vi "Upload File.vi"(8 "error in (no error)":errorcluster, 9 "Relative Path":string, 10 "Local File":path, 11 "Artifactory in":refnum<class "Artifactory.lvclass">) -> (0 "error out":errorcluster, 3 "Artifactory out":refnum<class "Artifactory.lvclass">)   [LabVIEW 2021, in "Artifactory.lvclass"]
uses:
  Artifactory.lvclass
  Actions -- enum.ctl
  Artifactory.lvclass/Artifactory.ctl
  <vilib>/addons/_JKI.lib/REST Client/classes/REST Client/REST Client.lvclass
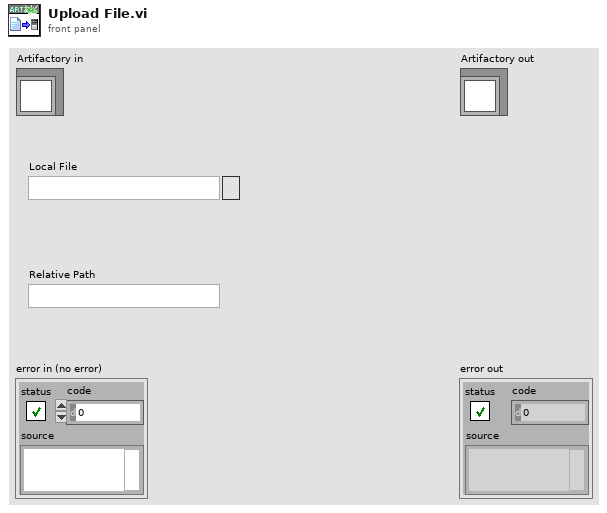
[diagram p1: front panel]
types:
  T1 = typedef "Artifactory.lvclass/Actions -- enum.ctl" = enum16{"Idle", "Custom Event", "Connecting to Artifactory", "Verifying Permissions", "Listing local repository", "Listing remote repository", "Computing changes", "Uploading file", "Downloading file"}
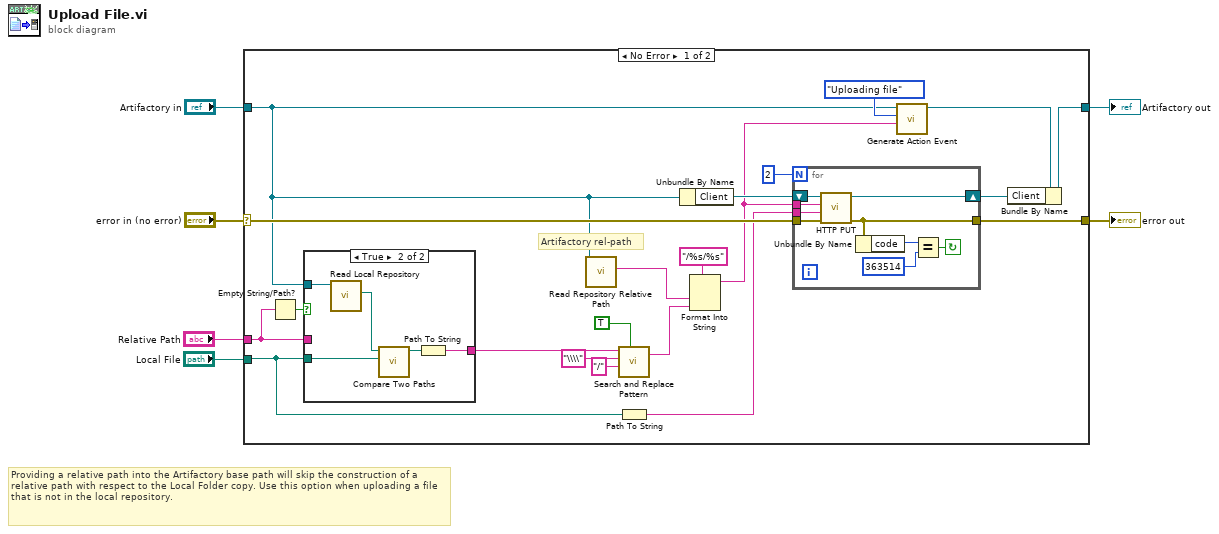
[diagram p0: block diagram]
diagram:
  # "Providing a relative path into the Artifactory base path will skip the construction of a relative path with respect to the Local Folder copy. Use this option when uploading a file that is not in the local repository."
  n1 = case shown="No Error" "error in (no error)" {
    selector: "error in (no error)" -> [w20 w44]
    tunnel: [w19 w44] -> w5
    tunnel: [w17 w43] -> w3
    tunnel: "Artifactory in" -> [w9 w43]
    tunnel: "Local File" -> [w12 _]
    tunnel: "Relative Path" -> [w7 _]
    frame No Error {
      # "Artifactory rel-path"
      n2 = Empty String/Path?(string/path=w7) -> (empty?=w8:bool)
      n3 = case shown="True" w8 {
        tunnel: [w28 w33] -> w25
        tunnel: w12 -> [_ w30]
        tunnel: w9 -> [_ w29]
        tunnel: w7 -> [w28 _]
        frame False {
        }
        frame True {
          n4 = call "Read Local Repository.vi"("Artifactory in"=w29) -> ("Local Repository"=w32:path)  [unwired: 9 in, 1 out]
          n5 = call <vilib>:"Compare Two Paths.vi"("Path 2"=w30, "Path 1"=w32) -> ("Relative Path from 1 to 2"=w31:path)  [unwired: 6 in, 3 out]
          n6 = Path To String(path=w31) -> (string=w33:string)
        }
      }
      n7 = call "Read Repository Relative Path.vi"("Artifactory in"=w9) -> ("repository path"=w15:string)  [unwired: 9 in, 1 out]
      n8 = call <vilib>:"Search and Replace Pattern.vi"("string"=w25, "regular expression (\"\")"="\\\\" ("regular expression (\"\")"), "replace string (\"\")"="/" ("regular expression (\"\")"), "replace all? (F)"=TRUE) -> ("result string"=w21:string)  [unwired: 1 in, 1 out]
      n9 = Path To String(path=w12) -> (string=w11:string)
      n10 = Unbundle By Name(w9) -> ("Client"=w26:refnum<class "REST Client.lvclass">)
      n11 = Format Into String(format string="/%s/%s" ("Path"), w15, w21) -> (resulting string=w10:string)  [unwired: 2 in, 1 out]
      n12 = for {
        N: 2 -> [_]
        tunnel: w10 -> [w41]
        tunnel: w11 -> [w39]
        shift-right: [w38] -> w18
        shift-left: w26 -> [w42]
        tunnel: w20 -> [w40]
        tunnel: [w37] -> w19
        stop <- w34 continue-if-true
        n13 = call-dynamic "HTTP PUT.vi"("error in (no error)"=w40, "Request body"=w39, "Path"=w41, "REST Client in"=w42) -> ("error out"=w37:errorcluster, "REST Client out"=w38:refnum<class "REST Client.lvclass">)  [unwired: 2 in, 4 out]
        n14 = Unbundle By Name(w37) -> ("code"=w36:i32)
        n15 = Equal?(x=w36, y=363514) -> (x = y?=w34:bool)
      }
      n16 = call-dynamic "Generate Action Event.vi"("Description"=w10, "Action"=Actions_--_enum."Uploading file", "Artifactory in"=w9) -> ("Artifactory out"=w13:refnum<class "Artifactory.lvclass">)  [unwired: 7 in, 1 out]
      n17 = Bundle By Name(cluster=w13, "Client"=w18) -> (w17:refnum<class "Artifactory.lvclass">)
    }
    frame Error {
    }
  }
  "error out" <- w5
  "Artifactory out" <- w3
